vi "Console Add.vi"(8 "Sender":T1, 11 "Data":string) -> ()   [LabVIEW 2018]
uses:
  Global variable.vi
  Typedef/Sender.ctl
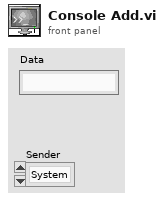
[diagram p1: front panel]
types:
  T1 = typedef "Sender.ctl" = enum16{"System", "Labview", "TCP", "User", "ORM", ""}
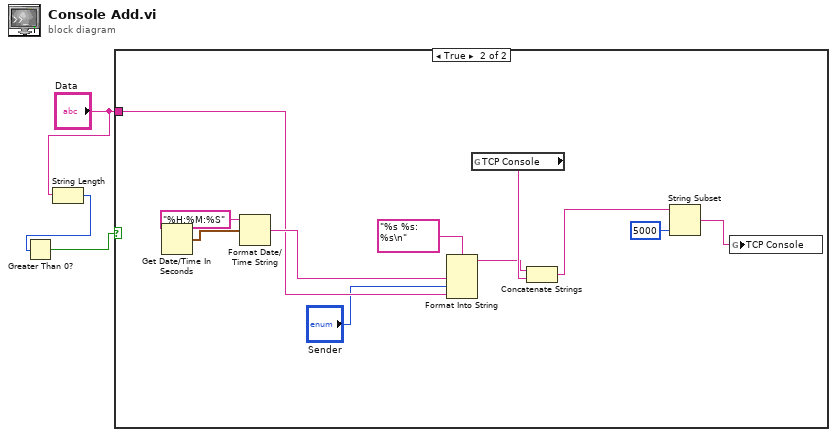
[diagram p0: block diagram]
diagram:
  n1 = String Length(string="Data") -> (length=w2:i32)
  n2 = Greater Than 0?(x=w2) -> (x > 0?=w3:bool)
  n3 = case shown="True" w3 {
    tunnel: "Data" -> [_ w10]
    frame False {
    }
    frame True {
      n4 = Get Date/Time In Seconds() -> (seconds since 1Jan1904=w14:timestamp)
      n5 = Format Date/Time String(time format string (%c)="%H:%M:%S", seconds (now)=w14) -> (date/time string=w11:string)  [unwired: 1 in]
      n6 = Format Into String(format string="%s %s: %s\n", w11, "Sender", w10) -> (resulting string=w5:string)  [unwired: 2 in, 1 out]
      n7 = global read "Global variable.vi" "TCP Console"() -> (w6:string)
      n8 = Concatenate Strings(w5, w6) -> (w8:string)
      n9 = String Subset(string=w8, length (rest)=5000 ("length (rest)")) -> (substring=w7:string)  [unwired: 1 in]
      n10 = global write "Global variable.vi" "TCP Console"(w7) -> ()
    }
  }
